vi "Sweep.Timed.vi"(4 "DataPoints":u64, 5 "frequency spacing":enum16{"Linear", "Logarithmic"}(ring)=enum."Logarithmic", 6 "Fsample (S/s)":dbl=44100.0 format="%^.2e", 7 "Offset":dbl=1.0 format="%.2f", 8 "error in (no error)":errorcluster, 9 "EndHz":dbl=10.0 format="%.2f", 10 "StartHz":dbl=1.0 format="%.2f", 11 "Amplitude":dbl=1.0 format="%.2f") -> (0 "error out":errorcluster, 3 "Chirp Data":dbl[](array[numeric]) format="%.5f")   [LabVIEW 2015, in "Single Station Execution.lvlib"]
uses:
  Single Station Execution.lvlib
  <vilib>/addons/_NISVFA/_Generation/SoundVib_Generation.lvlib
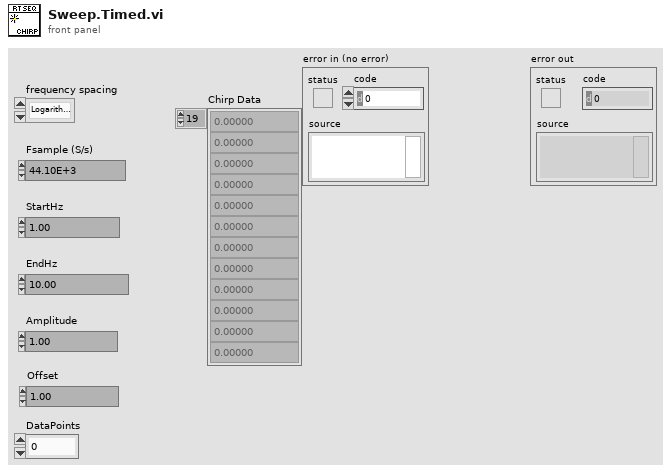
[diagram p1: front panel]
types:
  T1 = cluster{"start frequency [Hz]":dbl, "stop frequency [Hz]":dbl}
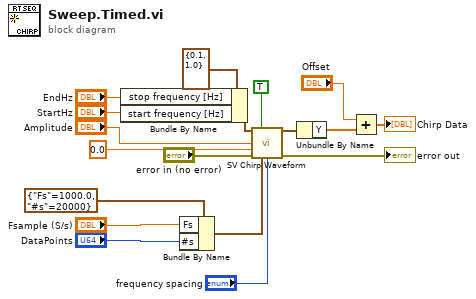
[diagram p0: block diagram]
diagram:
  n1 = Bundle By Name(cluster=T1 {"start frequency [Hz]"=0.1, "stop frequency [Hz]"=1.0} ("frequency range"), "stop frequency [Hz]"="EndHz", "start frequency [Hz]"="StartHz") -> (w4:T1)
  n2 = Bundle By Name(cluster=cluster{"Fs":dbl, "#s":u32} {"Fs"=1000.0, "#s"=20000} ("sampling info"), "Fs"="Fsample (S/s)", "#s"="DataPoints") -> (w7:cluster{"Fs":dbl, "#s":u32})
  n3 = call <vilib>:"SV Chirp Waveform.vi"("frequency range"=w4, "reset signal (F)"=TRUE, "amplitude"="Amplitude", "phase in [deg]"=0.0, "error in (no error)"="error in (no error)", "sampling info"=w7, "frequency spacing"="frequency spacing") -> ("chirp signal"=w10:waveform(dbl), "error out"=→"error out":errorcluster)  [unwired: 6 in, 1 out]
  n4 = Unbundle By Name(w10) -> ("Y"=w9:dbl[])
  n5 = Add(x="Offset", y=w9) -> (x+y=→"Chirp Data":dbl[])
